vi "Main.vi"() -> ()   [LabVIEW 2020, in "Example 1.lvlib"]
uses:
  Example 1.lvlib
  Scene/Scene.lvclass
  Scene/Mouse Button Held.ctl
  Graphics/Libraries/Utility/Utility.lvlib
panel:
  in  "Remove Active":bool
  in  "Add":bool
  in  "Turntable Enabled":bool
  out "Active Object":string
  in  "Alpha":dbl(slide) scale=0.0..1.0
  in  "Alpha Blending Enabled":bool
  in  "Diffuse Colour":u32(colorbox)
  out "Screen":picture
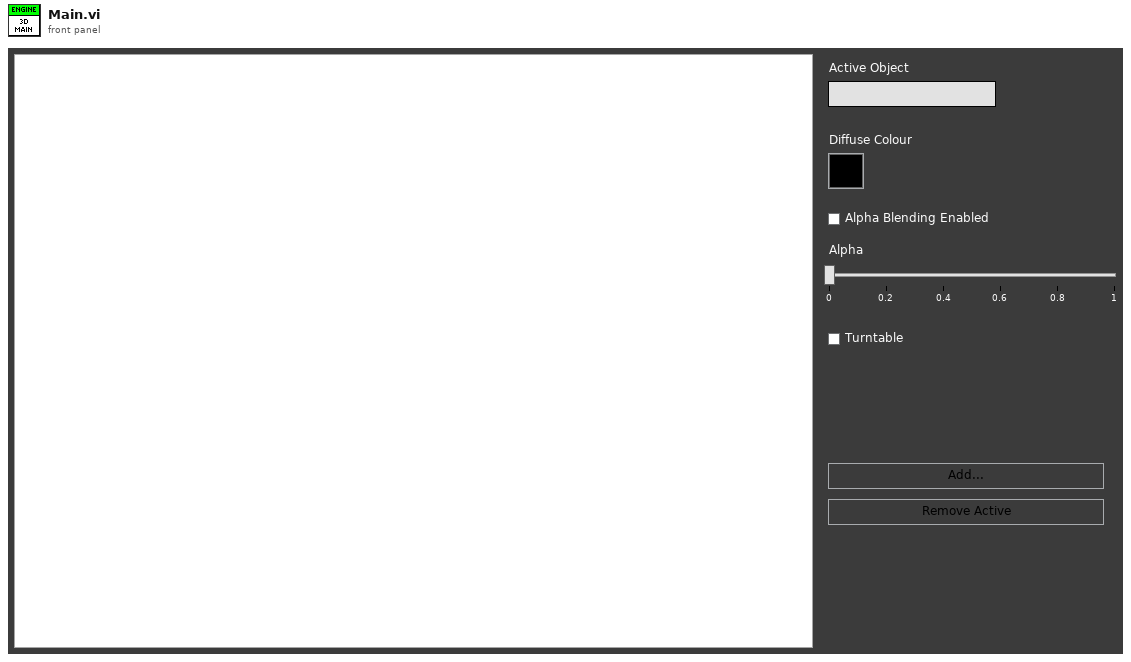
[diagram p1: front panel]
types:
  T1 = typedef "Example 1.lvlib/Core Data.ctl" = cluster{"Pixel Data":u32[][], "Scene":refnum<class "Scene.lvclass">, "Mouse Button Held":T2}
  T2 = typedef "Scene.lvclass/Mouse Button Held.ctl" = enum16{"None", "Left", "Middle", "Right"}
  T3 = enum32{"invalid app kind", "Development System", "Run Time System", "Student Edition", "Embedded LabVIEW", "Evaluation", "Custom"}
  T4 = typedef "Scene.lvclass/Camera Movement.ctl" = enum16{"Forward", "Backwards", "Up", "Down", "Left", "Right", "Yaw CCW", "Yaw CW"}
  T5 = typedef "LVPoint32TypeDef.ctl" = cluster{"Horizontal":i32, "Vertical":i32}
  T6 = typedef "3D.lvlib/Object.ctl" = cluster{"Triangles":T7[], "Transform":T14, "Name":string, "Alpha Blending Enabled":bool, "Alpha":dbl, "Turntable Enabled":bool, "Material":T11}
  T7 = typedef "3D.lvlib/Triangle.ctl" = cluster{"Vertex 1":T8, "Vertex 2":T8, "Vertex 3":T8, "Alpha":dbl, "Alpha Blending Enabled":bool, "Colour":u32, "Material":T11}
  T8 = typedef "3D.lvlib/Vertex.ctl" = cluster{"Position":T9, "UV":T10, "Colour":u32}
  T9 = typedef "3D.lvlib/Vector 3D.ctl" = cluster{"x":sgl, "y":sgl, "z":sgl}
  T10 = typedef "Raster.lvlib/UV.ctl" = cluster{"u":sgl, "v":sgl}
  T11 = typedef "3D.lvlib/Material.ctl" = cluster{"Diffuse Colour":u32, "Texture":T12}
  T12 = typedef "Raster.lvlib/Texture.ctl" = cluster{"Pixels":refnum<data-value>, "Size":T13}
  T13 = typedef "Raster.lvlib/Rectangle Dimensions.ctl" = cluster{"Width":u32, "Height":u32}
  T14 = typedef "3D.lvlib/Transform.ctl" = cluster{"Position":T9, "Rotation":T9, "Scale":T9}
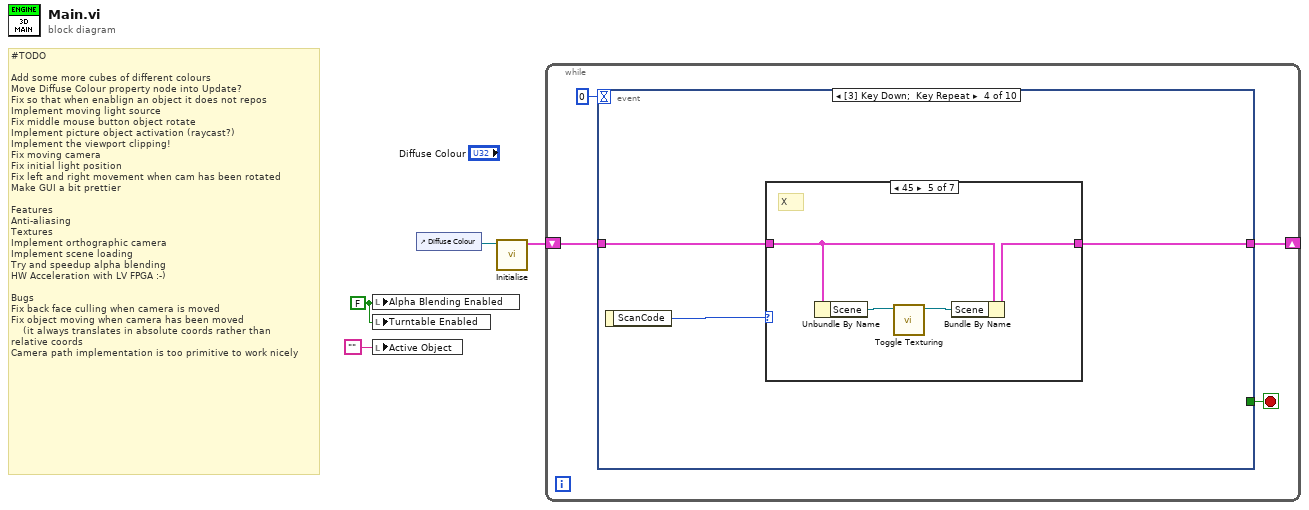
[diagram p0: block diagram]
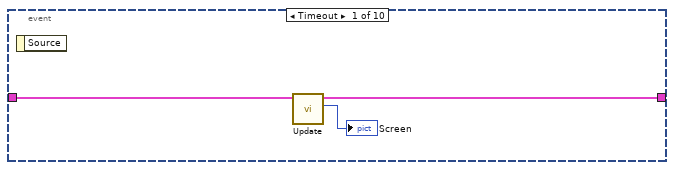
[diagram p2: hidden frame]
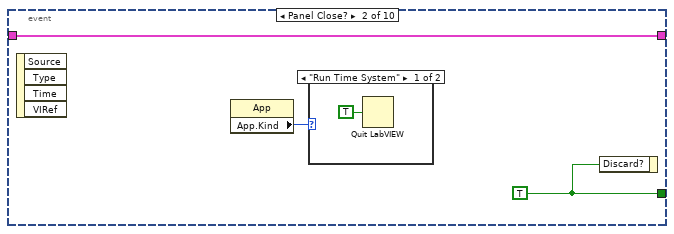
[diagram p3: hidden frame]
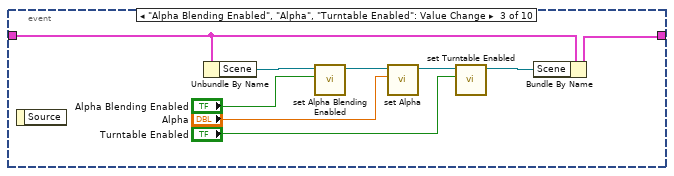
[diagram p5: hidden frame]
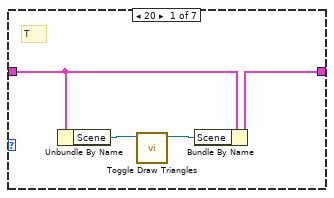
[diagram p6: hidden frame]
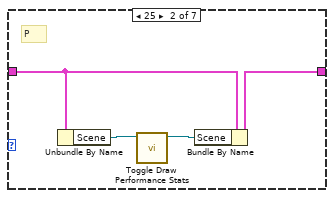
[diagram p7: hidden frame]
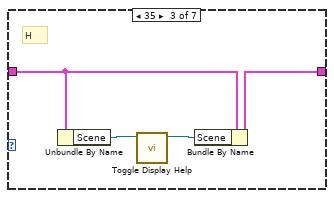
[diagram p8: hidden frame]
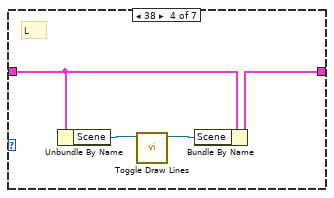
[diagram p9: hidden frame]
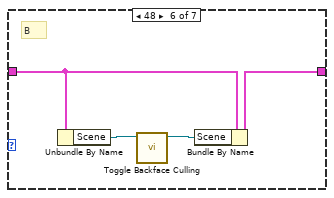
[diagram p10: hidden frame]
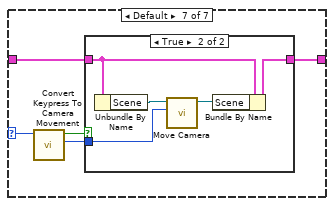
[diagram p11: hidden frame]
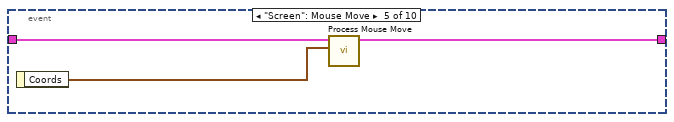
[diagram p13: hidden frame]
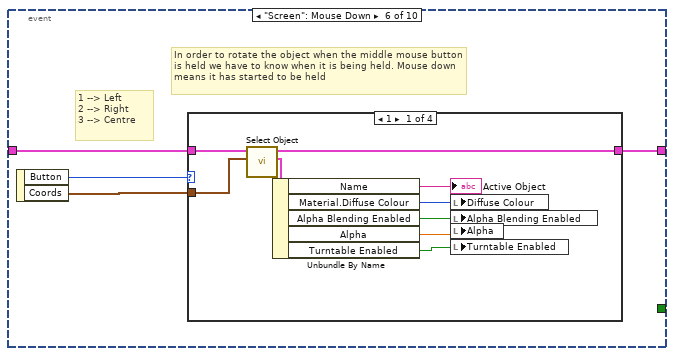
[diagram p14: hidden frame]
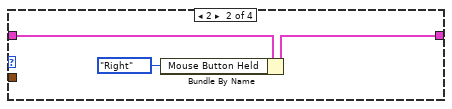
[diagram p15: hidden frame]
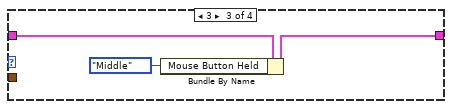
[diagram p16: hidden frame]
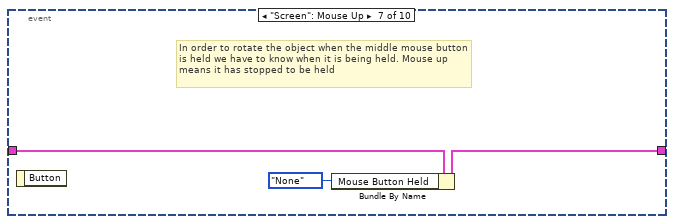
[diagram p18: hidden frame]
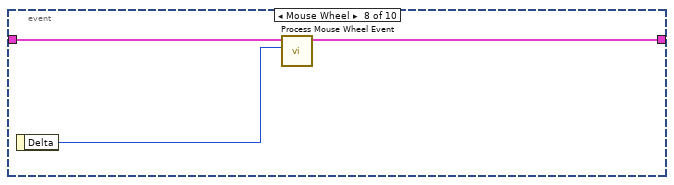
[diagram p19: hidden frame]
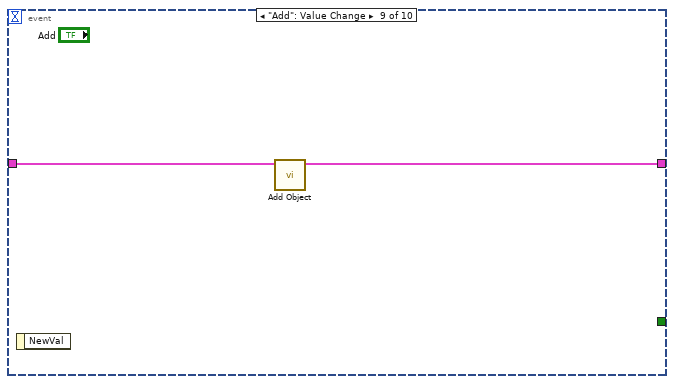
[diagram p20: hidden frame]
diagram:
  w2 = FALSE ("Enabled")
  # "#TODO\n\nAdd some more cubes of different colours\nMove Diffuse Colour property node into Update?\nFix so that when enablign an object it does not repos\nImplement moving light source\nFix middle mouse button object rotate\nImplement picture object activation (raycast?)\nImplement the viewport clipping!\nFix moving camera\nFix initial light position\nFix left and right movement when cam has been rotated\nMake GUI a bit prettier\n\nFeatures\nAnti-aliasing\nTextures\nImplement orthographic camera\nImplement scene loading\nTry and speedup alpha blending\nHW Acceleration with LV FPGA :-)\n\nBugs\nFix back face culling when camera is moved\nFix object moving when camera has been moved\n    (it always translates in absolute coords rather than                                                                                                      relative coords\nCamera path implementation is too primitive to work nicely"
  n1 = local write "Alpha Blending Enabled"(w2) -> ()
  n2 = local write "Turntable Enabled"(w2) -> ()
  n3 = local write "Active Object"("") -> ()
  n4 = control-ref of="Diffuse Colour"() -> (w3:refnum<vi>)
  n5 = call "Initialise.vi"("Diffuse Colour"=w3) -> ("Core Data out"=w4:T1)  [unwired: 10 in]
  n6 = while {
    shift-right: [w6] -> _
    shift-left: w4 -> [w7]
    stop <- w5 stop-if-true
    n7 = event shown="[3] Key Down;  Key Repeat" {
      selector: _ -> [_ _ _ _ _ _ _ _ _ _]
      dyn-events: _ -> [_ _ _ _ _ _ _ _ _ _]
      timeout: 0 -> [_ _ _ _ _ _ _ _ _ _]
      tunnel: w7 -> [w9 w14 w24 w27 w64 w68 w88 w90 w93 w95]
      tunnel: [w11 w14 w23 w26 w65 w67 w87 w91 w92 w94] -> w6
      tunnel: [_ w13 _ _ _ _ _ _ _ _] -> w5
      event Timeout {
        n8 = event-data() -> ()  [unwired: 1 in, 1 out]
        n9 = call "Update.vi"("Core Data in"=w9) -> ("Screen"=→"Screen":picture, "Core Data out"=w11:T1)  [unwired: 9 in]
      }
      event Panel Close? {
        w13 = TRUE ("Discard?")
        (unwired) TRUE ("Discard?")
        n10 = event-data() -> ()  [unwired: 1 in, 4 out]
        n11 = property class="App"() -> ("App.Kind"=w12:T3)  [unwired: 2 in, 2 out]
        n12 = case shown="\"Run Time System\"" w12 {
          frame "Run Time System" {
            n13 = Quit LabVIEW(quit? (T)=TRUE) -> ()
          }
          frame Default {
          }
        }
        n14 = event-data("Discard?"=w13) -> ()  [unwired: 1 in, 1 out]
      }
      event "Alpha Blending Enabled", "Alpha", "Turntable Enabled": Value Change {
        n15 = event-data() -> ()  [unwired: 1 in, 1 out]
        n16 = Unbundle By Name(w24) -> ("Scene"=w16:refnum<class "Scene.lvclass">)
        n17 = call "set Alpha Blending Enabled.vi"("Alpha Blending Enabled"="Alpha Blending Enabled", "Scene in"=w16) -> ("Scene out"=w22:refnum<class "Scene.lvclass">)  [unwired: 9 in]
        n18 = call "set Alpha.vi"("Alpha"="Alpha", "Scene in"=w22) -> ("Scene out"=w21:refnum<class "Scene.lvclass">)  [unwired: 9 in]
        n19 = call "set Turntable Enabled.vi"("Turntable Enabled"="Turntable Enabled", "Scene in"=w21) -> ("Scene out"=w20:refnum<class "Scene.lvclass">)  [unwired: 9 in]
        n20 = Bundle By Name(cluster=w24, "Scene"=w20) -> (w23:T1)
      }
      event Key Down; Key Repeat {
        n21 = event-data() -> ("ScanCode"=w25:i16)  [unwired: 1 in]
        n22 = case shown="45" w25 {
          selector: w25 -> [_ _ _ _ _ _ w54]
          tunnel: w27 -> [w30 w34 w38 w42 w46 w50 w56]
          tunnel: [w31 w35 w39 w43 w47 w51 w55] -> w26
          frame 20 {
            # "T"
            n23 = Unbundle By Name(w30) -> ("Scene"=w29:refnum<class "Scene.lvclass">)
            n24 = call "Toggle Draw Triangles.vi"("Scene in"=w29) -> ("Scene out"=w28:refnum<class "Scene.lvclass">)  [unwired: 10 in]
            n25 = Bundle By Name(cluster=w30, "Scene"=w28) -> (w31:T1)
          }
          frame 25 {
            # "P"
            n26 = Unbundle By Name(w34) -> ("Scene"=w33:refnum<class "Scene.lvclass">)
            n27 = call "Toggle Draw Performance Stats.vi"("Scene in"=w33) -> ("Scene out"=w32:refnum<class "Scene.lvclass">)  [unwired: 10 in]
            n28 = Bundle By Name(cluster=w34, "Scene"=w32) -> (w35:T1)
          }
          frame 35 {
            # "H"
            n29 = Unbundle By Name(w38) -> ("Scene"=w37:refnum<class "Scene.lvclass">)
            n30 = call "Toggle Display Help.vi"("Scene in"=w37) -> ("Scene out"=w36:refnum<class "Scene.lvclass">)  [unwired: 10 in]
            n31 = Bundle By Name(cluster=w38, "Scene"=w36) -> (w39:T1)
          }
          frame 38 {
            # "L"
            n32 = Unbundle By Name(w42) -> ("Scene"=w41:refnum<class "Scene.lvclass">)
            n33 = call "Toggle Draw Lines.vi"("Scene in"=w41) -> ("Scene out"=w40:refnum<class "Scene.lvclass">)  [unwired: 10 in]
            n34 = Bundle By Name(cluster=w42, "Scene"=w40) -> (w43:T1)
          }
          frame 45 {
            # "X"
            n35 = Unbundle By Name(w46) -> ("Scene"=w45:refnum<class "Scene.lvclass">)
            n36 = call "Toggle Texturing.vi"("Scene in"=w45) -> ("Scene out"=w44:refnum<class "Scene.lvclass">)  [unwired: 10 in]
            n37 = Bundle By Name(cluster=w46, "Scene"=w44) -> (w47:T1)
          }
          frame 48 {
            # "B"
            n38 = Unbundle By Name(w50) -> ("Scene"=w49:refnum<class "Scene.lvclass">)
            n39 = call "Toggle Backface Culling.vi"("Scene in"=w49) -> ("Scene out"=w48:refnum<class "Scene.lvclass">)  [unwired: 10 in]
            n40 = Bundle By Name(cluster=w50, "Scene"=w48) -> (w51:T1)
          }
          frame Default {
            n41 = call "Convert Keypress To Camera Movement.vi"("ScanCode"=w54) -> ("Camera Movement"=w52:T4, "Move Camera"=w53:bool)  [unwired: 9 in]
            n42 = case shown="True" w53 {
              tunnel: w56 -> [w57 w61]
              tunnel: [w57 w59] -> w55
              tunnel: w52 -> [_ w58]
              frame False {
              }
              frame True {
                n43 = Unbundle By Name(w61) -> ("Scene"=w62:refnum<class "Scene.lvclass">)
                n44 = call "Move Camera.vi"("Camera Movement"=w58, "Scene in"=w62) -> ("Scene out"=w60:refnum<class "Scene.lvclass">)  [unwired: 9 in]
                n45 = Bundle By Name(cluster=w61, "Scene"=w60) -> (w59:T1)
              }
            }
          }
        }
      }
      event "Screen": Mouse Move {
        n46 = event-data() -> ("Coords"=w63:T5)  [unwired: 1 in]
        n47 = call "Process Mouse Move.vi"("Coords"=w63, "Core Data in"=w64) -> ("Core Data out"=w65:T1)  [unwired: 9 in]
      }
      event "Screen": Mouse Down {
        # "1 --> Left\n2 --> Right\n3 --> Centre"
        # "In order to rotate the object when the middle mouse button is held we have to know when it is being held. Mouse down means it has started to be held"
        n48 = event-data() -> ("Button"=w69:u16, "Coords"=w66:T5)  [unwired: 1 in]
        n49 = case shown="1" w69 {
          tunnel: w68 -> [w78 w81 w84 w85]
          tunnel: [w77 w80 w83 w85] -> w67
          tunnel: w66 -> [w76 _ _ _]
          frame 1 {
            n50 = call "Select Object.vi"("Coords"=w76, "Core Data in"=w78) -> ("Object"=w75:T6, "Core Data out"=w77:T1)  [unwired: 8 in]
            n51 = Unbundle By Name(w75) -> ("Name"=→"Active Object":string, "Material.Diffuse Colour"=w74:u32, "Alpha Blending Enabled"=w72:bool, "Alpha"=w70:dbl, "Turntable Enabled"=w71:bool)
            n52 = local write "Diffuse Colour"(w74) -> ()
            n53 = local write "Alpha Blending Enabled"(w72) -> ()
            n54 = local write "Alpha"(w70) -> ()
            n55 = local write "Turntable Enabled"(w71) -> ()
          }
          frame 2 {
            n56 = Bundle By Name(cluster=w81, "Mouse Button Held"=Mouse_Button_Held."Right") -> (w80:T1)
          }
          frame 3 {
            n57 = Bundle By Name(cluster=w84, "Mouse Button Held"=Mouse_Button_Held."Middle") -> (w83:T1)
          }
          frame Default {
          }
        }
      }
      event "Screen": Mouse Up {
        # "In order to rotate the object when the middle mouse button is held we have to know when it is being held. Mouse up means it has stopped to be held"
        n58 = event-data() -> ()  [unwired: 1 in, 1 out]
        n59 = Bundle By Name(cluster=w88, "Mouse Button Held"=Mouse_Button_Held."None") -> (w87:T1)
      }
      event Mouse Wheel {
        n60 = event-data() -> ("Delta"=w89:i32)  [unwired: 1 in]
        n61 = call "Process Mouse Wheel Event.vi"("Delta"=w89, "Core Data in"=w90) -> ("Core Data out"=w91:T1)  [unwired: 9 in]
      }
      event "Add": Value Change {
        n62 = event-data() -> ()  [unwired: 1 in, 1 out]
        n63 = call "Add Object.vi"("Core Data in"=w93) -> ("Core Data out"=w92:T1)  [unwired: 10 in]
      }
      event "Remove Active": Value Change {
        n64 = event-data() -> ()  [unwired: 1 in, 3 out]
        n65 = call "Remove Active Object.vi"("Core Data in"=w95) -> ("Core Data out"=w94:T1)  [unwired: 10 in]
      }
    }
  }
